vi "Get Table Info.vi"(8 "error in":errorcluster, 11 "Connection in":refnum<k7>) -> (0 "error out":errorcluster, 2 "Info out":string[][](array[string]), 3 "Connection out":refnum<k7>)   [LabVIEW 2020, in "hse-db-ado.lvlib" / "ADO-DB-Driver.lvlib"]
doc: "Get table info\n\n____\nHAMPEL SOFTWARE ENGINEERING v1.4.0 (2023-12-19 09:52)"
uses:
  ADO-DB-Driver.lvlib
panel:
  # "TABLE_CATALOG      TABLE_SCHEMA       TABLE_NAME           TABLE_TYPE               TABLE_GUID            DESCRIPTION"
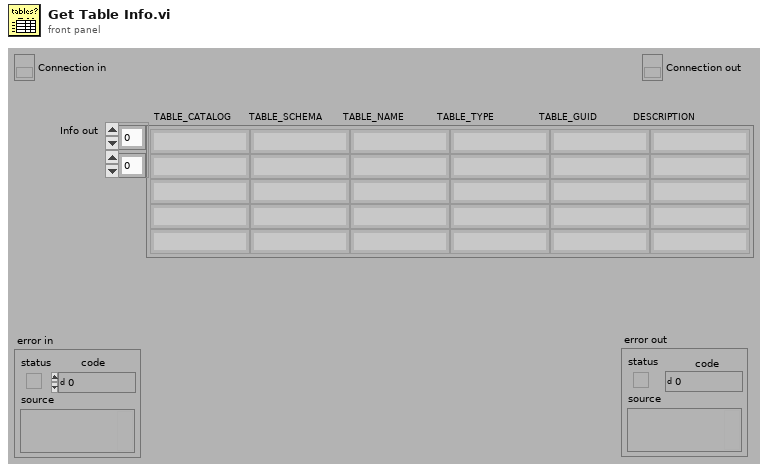
[diagram p1: front panel]
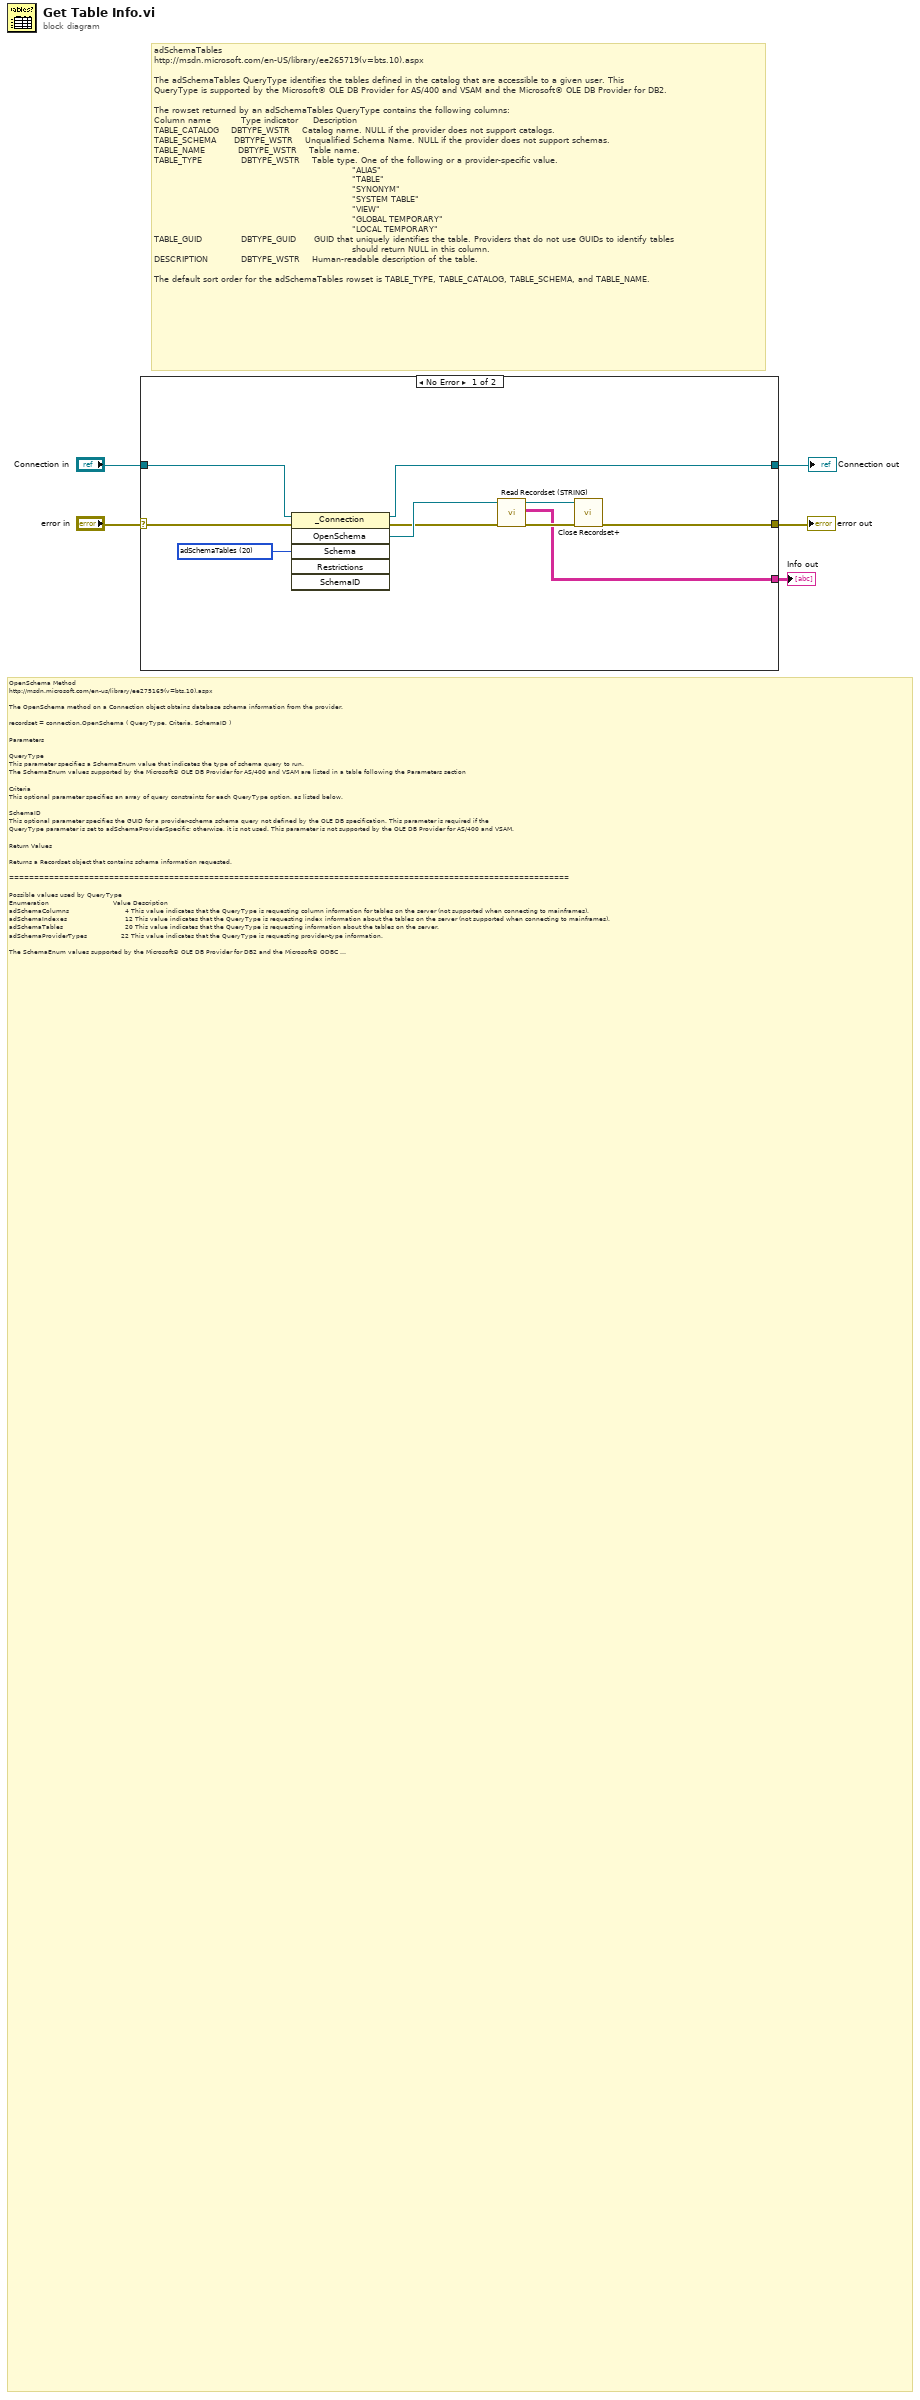
[diagram p0: block diagram]
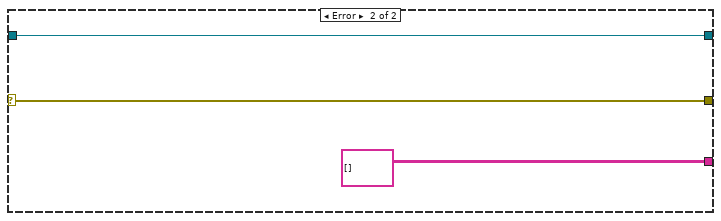
[diagram p2: hidden frame]
diagram:
  # "adSchemaTables\nhttp://msdn.microsoft.com/en-US/library/ee265719(v=bts.10).aspx\n\nThe adSchemaTables QueryType identifies the tables defined in the catalog that are accessible to a given user. This \nQueryType is supported by the Microsoft® OLE DB Provider for AS/400 and VSAM and the Microsoft® OLE DB Provider for DB2.\n\nThe rowset returned by an adSchemaTables QueryType contains the following columns:\nColumn name\t         Type indicator\t    Description\nTABLE_CATALOG\t   DBTYPE_WSTR\t   Catalog name. NULL if the provider does not support catalogs.\nTABLE_SCHEMA\t     DBTYPE_WSTR\t   Unqualified Schema Name. NULL if the provider does not support schemas.\nTABLE_NAME\t          DBTYPE_WSTR\t   Table name.\nTABLE_TYPE\t            DBTYPE_WSTR\t   Table type. One of the following or a provider-specific value.\n                                                                  \"ALIAS\"\n                                                                  \"TABLE\"\n                                                                  \"SYNONYM\"\n                                                                  \"SYSTEM TABLE\"\n                                                                  \"VIEW\"\n                                                                  \"GLOBAL TEMPORARY\"\n                                                                  \"LOCAL TEMPORARY\"\nTABLE_GUID\t            DBTYPE_GUID\t     GUID that uniquely identifies the table. Providers that do not use GUIDs to identify tables \n                                                                  should return NULL in this column.\nDESCRIPTION\t          DBTYPE_WSTR\t   Human-readable description of the table.\n\nThe default sort order for the adSchemaTables rowset is TABLE_TYPE, TABLE_CATALOG, TABLE_SCHEMA, and TABLE_NAME."
  # "OpenSchema Method\nhttp://msdn.microsoft.com/en-us/library/ee275169(v=bts.10).aspx\n\nThe OpenSchema method on a Connection object obtains database schema information from the provider.\n\nrecordset = connection.OpenSchema ( QueryType, Criteria, SchemaID )\n\nParameters\n\nQueryType\nThis parameter specifies a SchemaEnum value that indicates the type of schema query to run.\nThe SchemaEnum values supported by the Microsoft® OLE DB Provider for AS/400 and VSAM are listed in a table following the Parameters section\n\nCriteria\nThis optional parameter specifies an array of query constraints for each QueryType option, as listed below.\n\nSchemaID\nThis optional parameter specifies the GUID for a provider-schema schema query not defined by the OLE DB specification. This parameter is required if the \nQueryType parameter is set to adSchemaProviderSpecific; otherwise, it is not used. This parameter is not supported by the OLE DB Provider for AS/400 and VSAM.\n\nReturn Values\n\nReturns a Recordset object that contains schema information requested.\n\n================================================================================================================\n\nPossible values used by QueryType\nEnumeration\t                               Value\tDescription\nadSchemaColumns                           \t4\tThis value indicates that the QueryType is requesting column information for tables on the server (not supported when connecting to mainframes).\nadSchemaIndexes\t                            12\tThis value indicates that the QueryType is requesting index information about the tables on the server (not supported when connecting to mainframes).\nadSchemaTables\t                              20\tThis value indicates that the QueryType is requesting information about the tables on the server.\nadSchemaProviderTypes                 22\tThis value indicates that the QueryType is requesting provider-type information.\n\nThe SchemaEnum values supported by the Microsoft® OLE DB Provider for DB2 and the Microsoft® ODBC Driver for DB2 can be one of the following constants:\nEnumeration\t                                Value\tDescription\nadSchemaColumns\t                           4\tThis value indicates that the QueryType is requesting column information for tables on the server (not supported when connecting to mainframes).\nadSchemaIndexes\t                            12\tThis value indicates that the QueryType is requesting index information about the tables on the server (not supported when connecting to mainframes).\nadSchemaProcedures\t                     16\tThis value indicates that the QueryType is requesting information about stored procedures on the server.\nadSchemaTables                              \t20\tThis value indicates that the QueryType is requesting information about the tables on the server.\nadSchemaProviderTypes\t                22\tThis value indicates that the QueryType is requesting provider-type information.\nadSchemaProcedureParameters\t   26\tThis value indicates that the QueryType is requesting information about parameters used by stored procedures on the server.\nadSchemaPrimaryKeys\t                   28\tThis value indicates that the QueryType is requesting information about the primary keys for tables on the server.\n\nValues used by the Criteria parameter\nQueryType / Enumeration\nadSchemaColumns\nTABLE_CATALOG\nTABLE_SCHEMA\nTABLE_NAME\nCOLUMN_NAME\nadSchemaIndexes\nTABLE_CATALOG\nTABLE_SCHEMA\nINDEX_NAME\nTYPE\nTABLE_NAME\nadSchemaTables\nTABLE_CATALOG\nTABLE_SCHEMA\nTABLE_NAME\nTABLE_TYPE\nadSchemaProviderTypes\nDATA_TYPE\nBEST_MATCH\nThe values supported by the OLE DB Provider for DB2 and the ODBC Driver for DB2 can be one of the following constants depending on the QueryType:\nQueryType / Enumeration\nadSchemaColumns\nTABLE_CATALOG\nTABLE_SCHEMA\nTABLE_NAME\nCOLUMN_NAME\nadSchemaIndexes\nTABLE_CATALOG\nTABLE_SCHEMA\nINDEX_NAME\nTABLE_NAME\nadSchemaPrimaryKeys\nTABLE_CATALOG\nTABLE_SCHEMA\nTABLE_NAME\nadSchemaProcedures\nPROCEDURE_CATALOG\nPROCEDURE_SCHEMA (see Notes)\nPROCEDURE_NAME\nPROCEDURE_TYPE\nadSchemaProcedureParameters\nPROCEDURE_CATALOG\nPROCEDURE_SCHEMA (see Notes)\nPROCEDURE_NAME\nPROCEDURE_TYPE\nadSchemaProviderTypes\nDATA_TYPE\nBEST_MATCH\nadSchemaTables\nTABLE_CATALOG\nTABLE_SCHEMA\nTABLE_NAME\nTABLE_TYPE\n\n================================================================================================================\n\nRemarks\n\nThe OpenSchema method on a Connection object is used to return information about the data source, such as information about the tables on the server and the columns \nin the tables.\n\nThe Criteria argument is an array of values that can be used to limit the results of a schema query. Each schema query supports a different set of parameters. The actual \nschemas are defined by the OLE DB specification under the IDBSchemaRowset interface. The schema queries supported in ADO 1.5 and later by the OLE DB Provider for \nAS/400 and VSAM are listed above.\n\nThe OpenSchema method allows an application to pass at run time the target library of a Partioned Data Set (PDS/PDSE), a dataset, or a member name as one of the Criteria \narray arguments to retrieve the schema.\n\nProviders are not required to support all of the OLE DB standard schema QueryType values. Specifically, only adSchemaTables, adSchemaColumns, and \nadSchemaProviderTypes are required by the OLE DB specification. However, the provider is not required to support the Criteria constraints listed above for those schema \nqueries. Support for other schema QueryType values is optional.\n\nThe schema information specified in OLE DB is based on the assumption that providers support the concepts of a catalog and a schema. The ANSI SQL 92 specification \ndefines them as follows:\n- A catalog contains one or more schemas, but always contains a schema named INFORMATION_SCHEMA which contains the views and domains of the information \n   schema. In Microsoft® SQL Server and Microsoft® Access terms, a catalog is a database; in ODBC 2.x terms, a catalog is a qualifier.\n- A schema is a collection of database objects that are owned or have been created by a particular user. In Microsoft SQL Server and ODBC 2.x terms, a schema is an owner; \n   there is no equivalent to a schema in a Microsoft Access database.\n\nSchema information in ADO and OLE DB is retrieved using predefined schema rowsets. The following section lists the contents of each schema rowset supported by the \nOLE DB Provider for AS/400 and VSAM or the OLE DB Provider for DB2."
  n1 = case shown="No Error" "error in" {
    selector: "error in" -> [w14 w18]
    tunnel: [w12 w17] -> w5
    tunnel: [w7 w18] -> w4
    tunnel: "Connection in" -> [w13 w17]
    tunnel: [w6 string[][] [] ("Data out")] -> w1
    frame No Error {
      w15 = 20 items=["adSchemaProviderSpecific"=-1, "adSchemaAsserts"=0, "adSchemaCatalogs"=1, "adSchemaCharacterSets"=2, "adSchemaCollations"=3, "adSchemaColumns"=4, "adSchemaCheckConstraints"=5, "adSchemaConstraintColumnUsage"=6, "adSchemaConstraintTableUsage"=7, "adSchemaKeyColumnUsage"=8, "adSchemaReferentialContraints, adSchemaReferentialConstraints"=9, "adSchemaTableConstraints"=10, "adSchemaColumnsDomainUsage"=11, "adSchemaIndexes"=12, "adSchemaColumnPrivileges"=13, "adSchemaTablePrivileges"=14, "adSchemaUsagePrivileges"=15, "adSchemaProcedures"=16, "adSchemaSchemata"=17, "adSchemaSQLLanguages"=18, "adSchemaStatistics"=19, "adSchemaTables"=20, "adSchemaTranslations"=21, "adSchemaProviderTypes"=22, "adSchemaViews"=23, "adSchemaViewColumnUsage"=24, "adSchemaViewTableUsage"=25, "adSchemaProcedureParameters"=26, "adSchemaForeignKeys"=27, "adSchemaPrimaryKeys"=28, "adSchemaProcedureColumns"=29, "adSchemaDBInfoKeywords"=30, "adSchemaDBInfoLiterals"=31, "adSchemaCubes"=32, "adSchemaDimensions"=33, "adSchemaHierarchies"=34, "adSchemaLevels"=35, "adSchemaMeasures"=36, "adSchemaProperties"=37, "adSchemaMembers"=38, "adSchemaTrustees"=39] ("Schema")
      n2 = invoke class="_Connection" method="OpenSchema"(reference=w13, error in=w14, "Schema"=w15) -> (reference out=w12:refnum<k7>, error out=w10:errorcluster, "OpenSchema"=w11:refnum<k7>)  [unwired: 3 in, 3 out]
      n3 = call "Read Recordset (STRING).vi"("error in (no error)"=w10, "Recordset In"=w11) -> ("error out"=w9:errorcluster, "Data out"=w6:string[][], "Recordset Out"=w8:refnum<k7>)  [unwired: 5 in, 2 out]
      n4 = call "Close Recordset+.vi"("error in"=w9, "Recordset"=w8) -> ("error out"=w7:errorcluster)  [unwired: 9 in]
    }
    frame Error {
    }
  }
  "error out" <- w4
  "Connection out" <- w5
  "Info out" <- w1
